vi "CCE RRMA P04 SubVI03.vi"(9 "Cy":u32, 10 "Cx":u32, 11 "imagen":u32[][](array[numeric])) -> (3 "firma":dbl[](array[numeric]))   [LabVIEW 2020]
doc: "Ceballos Conde Emanuel Rodríguez Ramírez Miguel Ángel 4MV6 Sistemas de visión artificial 2022/1\nEste vi permite obtener la firma de una imagen en formato png con el contorno de 1 pixel de grosor"
panel:
  # "Ceballos Conde Emanuel\nRodríguez Ramírez Miguel Ángel\n4MV6\nSistemas de visión artificial\n2022/1"
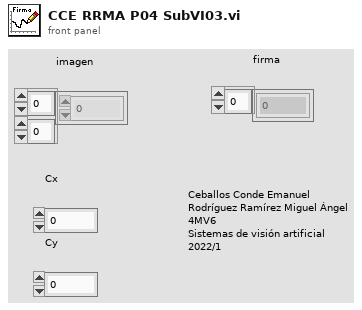
[diagram p1: front panel]
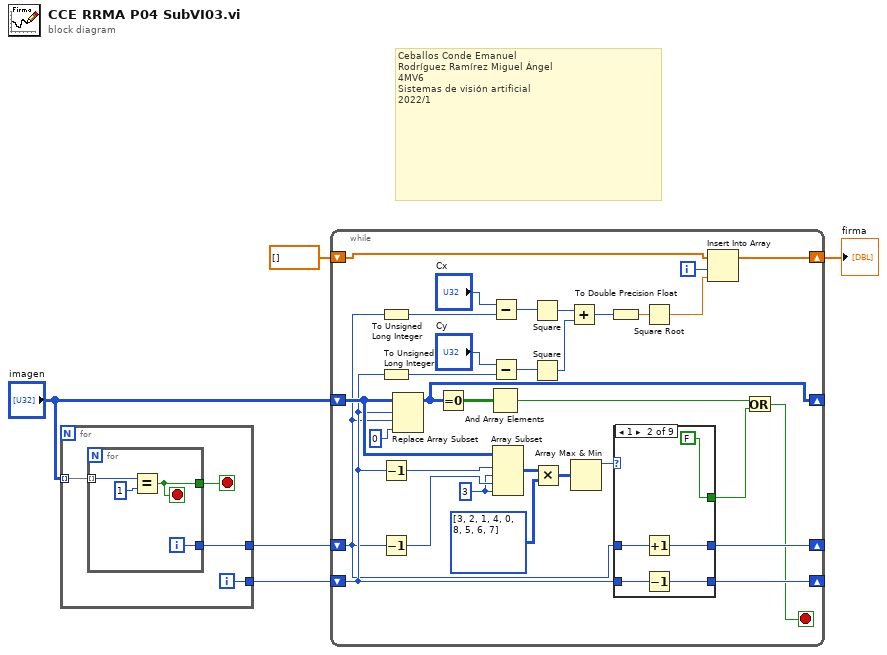
[diagram p0: block diagram]
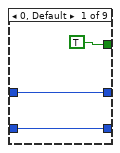
[diagram p2: hidden frame]
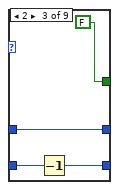
[diagram p3: hidden frame]
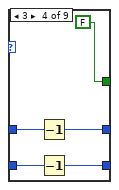
[diagram p4: hidden frame]
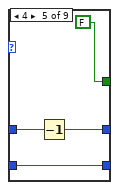
[diagram p5: hidden frame]
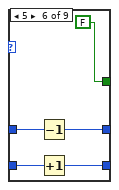
[diagram p6: hidden frame]
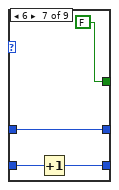
[diagram p7: hidden frame]
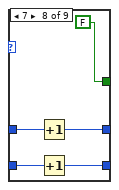
[diagram p8: hidden frame]
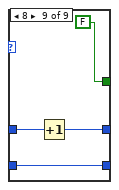
[diagram p9: hidden frame]
diagram:
  # "Ceballos Conde Emanuel\nRodríguez Ramírez Miguel Ángel\n4MV6\nSistemas de visión artificial\n2022/1"
  n1 = for {
    tunnel: "imagen" -> [w9] mode=indexing
    tunnel: [w7] -> w4
    tunnel: [w6] -> w3
    i -> [w6]
    stop <- w8 stop-if-true
    n2 = for {
      tunnel: w9 -> [w13] mode=indexing
      tunnel: [w11] -> w8
      tunnel: [w10] -> w7
      i -> [w10]
      stop <- w11 stop-if-true
      n3 = Equal?(x=w13, y=u32 1) -> (x = y?=w11:bool)
    }
  }
  n4 = while {
    shift-right: [w26] -> _
    shift-left: w4 -> [w22]
    shift-right: [w25] -> _
    shift-left: w3 -> [w23]
    shift-right: [w30] -> w2
    shift-left: dbl[] [] -> [w29]
    shift-right: [w14] -> _
    shift-left: "imagen" -> [w24]
    i -> [w28]
    stop <- w16 stop-if-true
    w43 = 3 ("length")
    n5 = To Unsigned Long Integer(number=w22) -> (unsigned 32bit integer=w18:u32)
    n6 = To Unsigned Long Integer(number=w23) -> (unsigned 32bit integer=w17:u32)
    n7 = Decrement(x=w23) -> (x-1=w45:i32)
    n8 = Decrement(x=w22) -> (x-1=w44:i32)
    n9 = Replace Array Subset(array=w24, new element=u32 0 ("new element/subarray"), index (row)=w23, index (col)=w22) -> (w14:u32[][])
    n10 = Equal To 0?(x=w14) -> (x = 0?=w20:bool[][])
    n11 = And Array Elements(Boolean array=w20) -> (logical AND=w19:bool)
    n12 = Subtract(x="Cx", y=w18) -> (x-y=w37:u32)
    n13 = Subtract(x="Cy", y=w17) -> (x-y=w34:u32)
    n14 = Array Subset(array=w24, index (row)=w45, length (row)=w43, index (col)=w44, length (col)=w43) -> (w42:u32[][])
    n15 = Square(x=w37) -> (x^2=w35:u32)
    n16 = Square(x=w34) -> (x^2=w33:u32)
    n17 = Multiply(x=w42, y=u32[][] [[3, 2, 1], [4, 0, 8], [5, 6, 7]]) -> (x*y=w40:u32[][])
    n18 = Add(x=w35, y=w33) -> (x+y=w36:u32)
    n19 = Array Max & Min(array=w40) -> (max value=w39:u32)  [unwired: 3 out]
    n20 = To Double Precision Float(number=w36) -> (double precision float=w31:dbl)
    n21 = case shown="1" w39 {
      tunnel: w23 -> [w47 w50 w56 w59 w66 w68 w74 w78 w84]
      tunnel: w22 -> [w48 w51 w57 w62 w65 w71 w75 w80 w83]
      tunnel: [w48 w53 w57 w61 w64 w70 w75 w79 w82] -> w26
      tunnel: [w47 w52 w55 w60 w66 w69 w73 w77 w84] -> w25
      tunnel: [TRUE FALSE FALSE FALSE FALSE FALSE FALSE FALSE FALSE] -> w15
      frame 0, Default {
      }
      frame 1 {
        n22 = Increment(x=w51) -> (x+1=w53:i32)
        n23 = Decrement(x=w50) -> (x-1=w52:i32)
      }
      frame 2 {
        n24 = Decrement(x=w56) -> (x-1=w55:i32)
      }
      frame 3 {
        n25 = Decrement(x=w62) -> (x-1=w61:i32)
        n26 = Decrement(x=w59) -> (x-1=w60:i32)
      }
      frame 4 {
        n27 = Decrement(x=w65) -> (x-1=w64:i32)
      }
      frame 5 {
        n28 = Decrement(x=w71) -> (x-1=w70:i32)
        n29 = Increment(x=w68) -> (x+1=w69:i32)
      }
      frame 6 {
        n30 = Increment(x=w74) -> (x+1=w73:i32)
      }
      frame 7 {
        n31 = Increment(x=w80) -> (x+1=w79:i32)
        n32 = Increment(x=w78) -> (x+1=w77:i32)
      }
      frame 8 {
        n33 = Increment(x=w83) -> (x+1=w82:i32)
      }
    }
    n34 = Square Root(x=w31) -> (sqrt(x)=w27:dbl)
    n35 = Insert Into Array(array=w29, index=w28, new element=w27) -> (w30:dbl[])
    n36 = Or(x=w19, y=w15) -> (x .or. y?=w16:bool)
  }
  "firma" <- w2
